vi "Autocalc Octree resolution.vi"(1 "Triangles array":T1[](array[typedef])) -> (0 "Suggested resolution":sgl)   [LabVIEW 2014]
uses:
  Typedefs/Triangle.ctl
panel:
  in  "Max branch level":i32=5
  # "PN 20/01/2015, 28/08/2015 (max branch level)"
  # "Vertices"
  # "Edges"
  # "Unit normal"
  # "Edge unit normals"
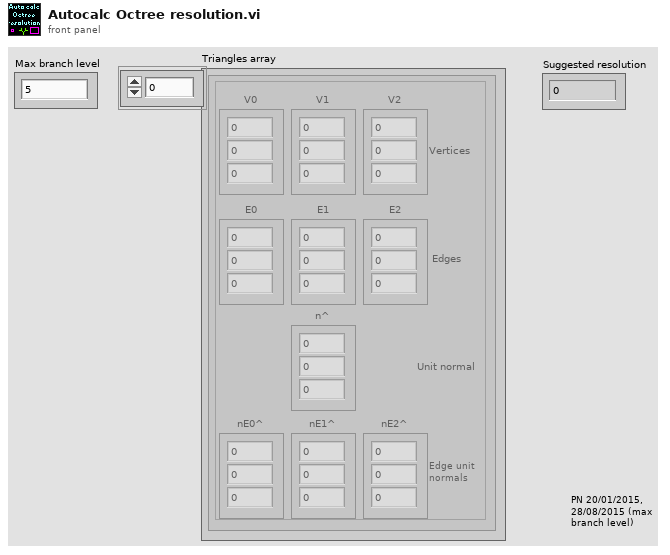
[diagram p1: front panel]
types:
  T1 = typedef "Triangle.ctl" = cluster{"V0":sgl[], "V1":sgl[], "V2":sgl[], "E0":sgl[], "E1":sgl[], "E2":sgl[], "n^":sgl[], "nE0^":sgl[], "nE1^":sgl[], "nE2^":sgl[]}
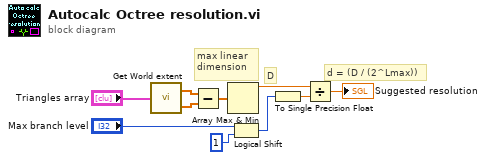
[diagram p0: block diagram]
diagram:
  # "d = (D / (2^Lmax))"
  # "D"
  # "max linear dimension"
  n1 = call "Get World extent.vi"("Triangles"="Triangles array") -> ("Pmax (x, y, z)"=w7:sgl[], "Pmin (x, y, z)"=w6:sgl[])
  n2 = Subtract(x=w7, y=w6) -> (x-y=w9:sgl[])
  n3 = Array Max & Min(array=w9) -> (max value=w8:sgl)  [unwired: 3 out]
  n4 = Logical Shift(y="Max branch level", x=u32 1) -> (x << y=w3:u32)
  n5 = To Single Precision Float(number=w3) -> (single precision float=w2:sgl)
  n6 = Divide(x=w8, y=w2) -> (x/y=→"Suggested resolution":sgl)
